vi "XML Find XML Expression.vi"(7 "Data Type":T1, 8 "error in (no error)":errorcluster, 10 "XPath expression":string, 11 "Refnum in":refnum<k20>) -> (0 "error out":errorcluster, 2 "Expressions":string[](array[string]), 3 "Refnum out":refnum<k20>)   [LabVIEW 2014]
uses:
  Type Definitions/XML Data Type.ctl
  <vilib>/xml/NI_XML.lvlib
  <resource>/objmgr/DOMUserDefRef.rc
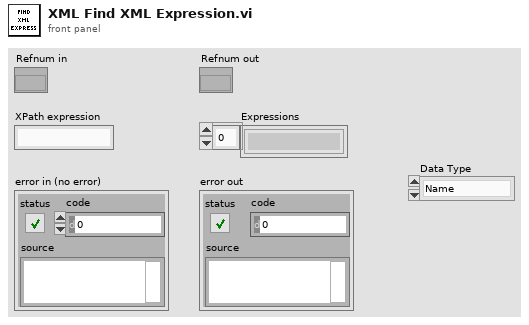
[diagram p1: front panel]
types:
  T1 = typedef "XML Data Type.ctl" = enum16{"Name", "Value"}
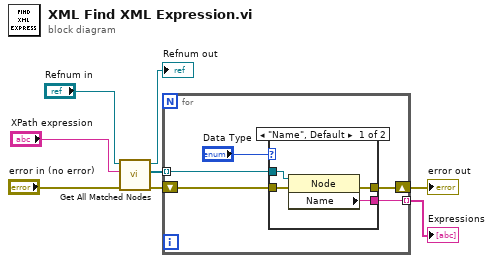
[diagram p0: block diagram]
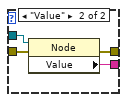
[diagram p2: hidden frame]
diagram:
  n1 = call <vilib>:"Get All Matched Nodes.vi"("error in (no error)"="error in (no error)", "XPath expression"="XPath expression", "node in"="Refnum in") -> ("error out"=w4:errorcluster, "node result array"=w2:refnum<k20>[], "node out"=→"Refnum out":refnum<k20>)  [unwired: 6 in]
  n2 = for {
    tunnel: w2 -> [w13] mode=indexing
    tunnel: [w12] -> w3 mode=indexing
    shift-right: [w11] -> w8
    shift-left: w4 -> [w10]
    n3 = case shown="\"Name\", Default" "Data Type" {
      tunnel: w13 -> [w17 w21]
      tunnel: [w16 w19] -> w12
      tunnel: [w15 w20] -> w11
      tunnel: w10 -> [w14 w18]
      frame "Name", Default {
        n4 = property class="Node"(reference=w17, error in=w14) -> (error out=w15:errorcluster, "Name"=w16:string)  [unwired: 1 out]
      }
      frame "Value" {
        n5 = property class="Node"(reference=w21, error in=w18) -> (error out=w20:errorcluster, "Value"=w19:string)  [unwired: 1 out]
      }
    }
  }
  "error out" <- w8
  "Expressions" <- w3
